vi "ErrorCheckHWI.vi"(8 "error in (no error)":errorcluster, 11 "NI Card in":refnum<class "NI Card.lvclass">) -> (0 "error out":errorcluster, 3 "NI Card out":refnum<class "NI Card.lvclass">)   [LabVIEW 2013, in "NI Card.lvclass"]
uses:
  NI Card.lvclass
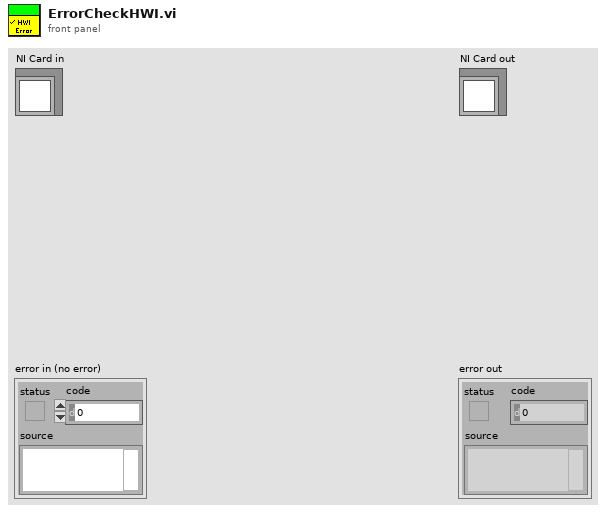
[diagram p1: front panel]
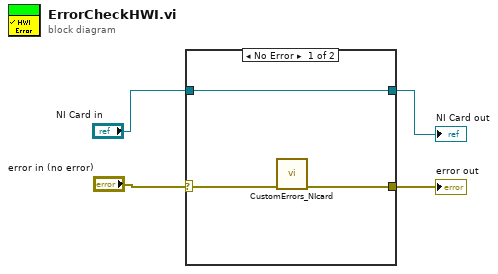
[diagram p0: block diagram]
diagram:
  n1 = case shown="No Error" "error in (no error)" {
    selector: "error in (no error)" -> [w6 w9]
    tunnel: "NI Card in" -> [w7 w8]
    tunnel: [w7 w8] -> w2
    tunnel: [w5 w9] -> w1
    frame No Error {
      n2 = call "CustomErrors_NIcard.vi"("error in (no error)"=w6) -> ("error out"=w5:errorcluster)  [unwired: 10 in]
    }
    frame Error {
    }
  }
  "error out" <- w1
  "NI Card out" <- w2
